vi "Add Library To Project.vi"(8 "error in":errorcluster, 10 "template folder path":path, 11 "configuration":T1) -> (0 "error out":errorcluster, 3 "project ref out":refnum<vi>)   [LabVIEW 2021, in "InstrumentStudio Plug-In Editor.lvlib"]
uses:
  InstrumentStudio Plug-In Editor.lvlib
  controls/Data Holder.ctl
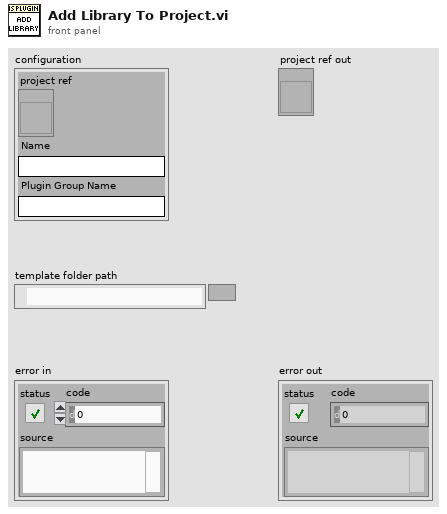
[diagram p1: front panel]
types:
  T1 = typedef "InstrumentStudio Plug-In Editor.lvlib/Data Holder.ctl" = cluster{"project ref":refnum<vi>, "Name":string, "Plugin Group Name":string}
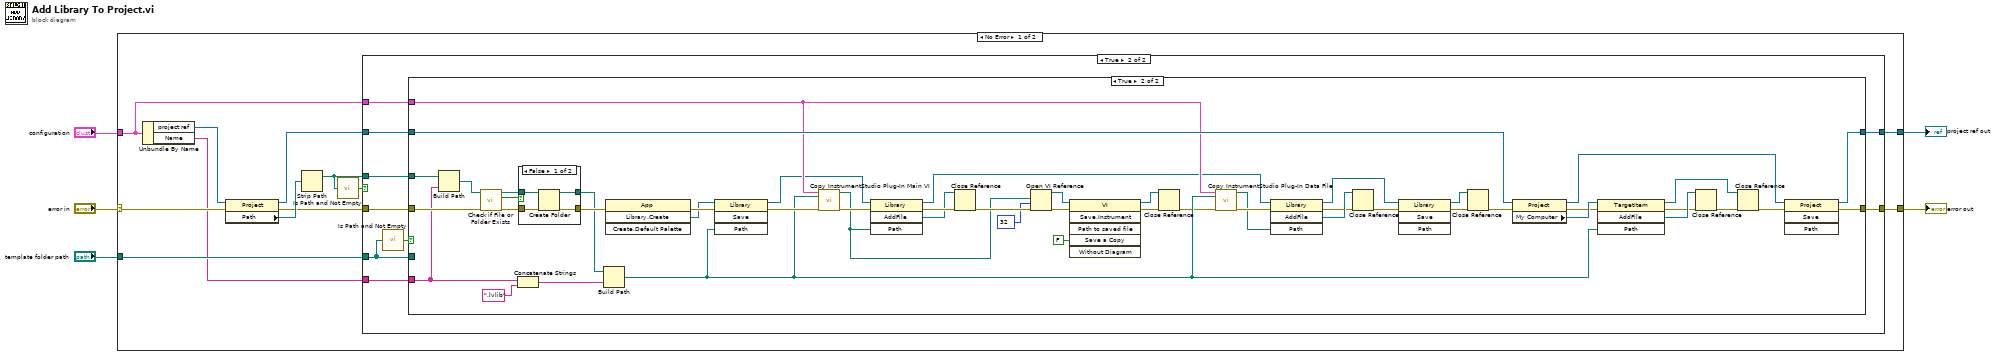
[diagram p0: block diagram]
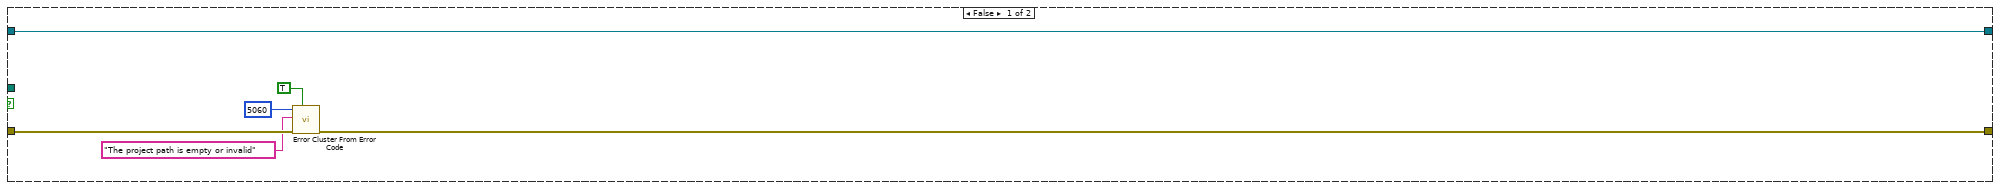
[diagram p2: hidden frame]
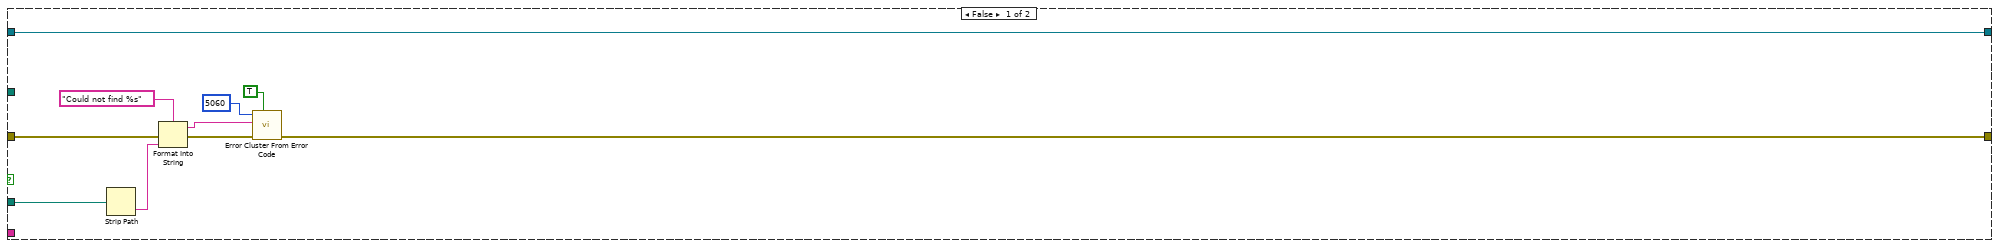
[diagram p3: hidden frame]
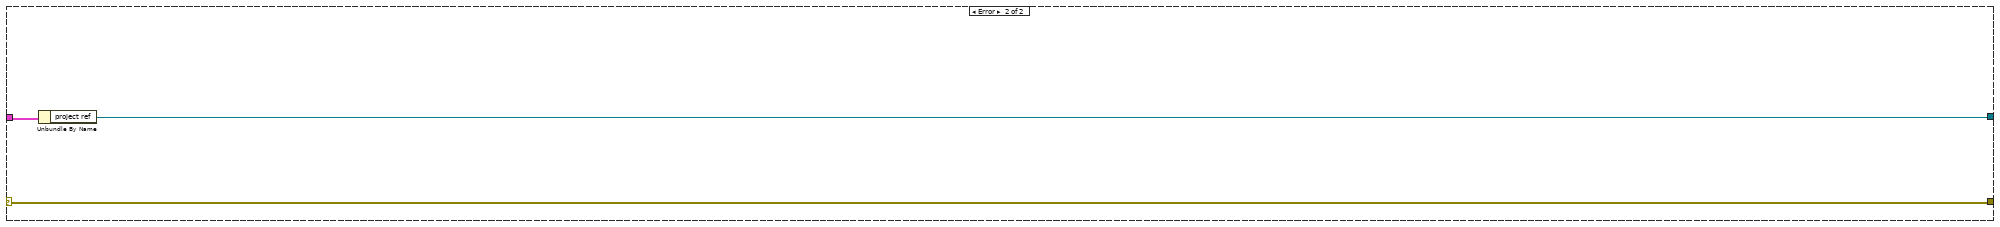
[diagram p5: hidden frame]
diagram:
  n1 = case shown="No Error" "error in" {
    selector: "error in" -> [w10 w100]
    tunnel: "template folder path" -> [w15 _]
    tunnel: [w14 w101] -> w5
    tunnel: "configuration" -> [w12 w99]
    tunnel: [w8 w100] -> w4
    frame No Error {
      n2 = Unbundle By Name(w12) -> ("project ref"=w13:refnum<vi>, "Name"=w6:string)
      n3 = property class="Project"(reference=w13, error in=w10) -> (reference out=w11:refnum<vi>, error out=w9:errorcluster, "Path"=w16:path)
      n4 = Strip Path(path=w16) -> (stripped path=w7:path)  [unwired: 1 out]
      n5 = call <vilib>:"Is Path and Not Empty.vi"("path"=w7) -> ("Is Path and Not Empty?"=w17:bool)  [unwired: 4 in]
      n6 = case shown="True" w17 {
        tunnel: w15 -> [_ w24]
        tunnel: w6 -> [_ w32]
        tunnel: w7 -> [_ w31]
        tunnel: [w23 w30] -> w14
        tunnel: w12 -> [_ w29]
        tunnel: w11 -> [w23 w28]
        tunnel: w9 -> [w22 w26]
        tunnel: [w18 w25] -> w8
        frame False {
          n7 = call <vilib>:"Error Cluster From Error Code.vi"("show call chain? (False)"=TRUE, "error in (no error)"=w22, "error message (\"\")"="The project path is empty or invalid" ("error message (\"\")"), "error code (0)"=5060) -> ("error out"=w18:errorcluster)  [unwired: 5 in]
        }
        frame True {
          n8 = call <vilib>:"Is Path and Not Empty.vi"("path"=w24) -> ("Is Path and Not Empty?"=w27:bool)  [unwired: 4 in]
          n9 = case shown="True" w27 {
            tunnel: w24 -> [w33 _]
            tunnel: w32 -> [_ w63]
            tunnel: w31 -> [_ w92]
            tunnel: [w40 w90] -> w30
            tunnel: w29 -> [_ w58]
            tunnel: w28 -> [w40 w69]
            tunnel: w26 -> [w37 w88]
            tunnel: [w34 w65] -> w25
            frame False {
              n10 = Strip Path(path=w33) -> (name=w38:string)  [unwired: 1 out]
              n11 = Format Into String(format string="Could not find %s", error in=w37, w38) -> (resulting string=w41:string, error out=w42:errorcluster)  [unwired: 1 in]
              n12 = call <vilib>:"Error Cluster From Error Code.vi"("show call chain? (False)"=TRUE, "error in (no error)"=w42, "error message (\"\")"=w41, "error code (0)"=5060) -> ("error out"=w34:errorcluster)  [unwired: 5 in]
            }
            frame True {
              n13 = Build Path(base path=w92, name or relative path=w63) -> (appended path=w91:path)
              n14 = call <vilib>:"Check if File or Folder Exists.vi"("error in (no error)"=w88, "path"=w91) -> ("error out"=w87:errorcluster, "file or folder exists?"=w85:bool, "dup path"=w86:path)  [unwired: 7 in]
              n15 = Concatenate Strings(w63, ".lvlib" ("string")) -> (w61:string)
              n16 = case shown="False" w85 {
                tunnel: w87 -> [w96 w97]
                tunnel: w86 -> [w95 w98]
                tunnel: [w94 w98] -> w62
                tunnel: [w93 w97] -> w84
                frame False {
                  n17 = Create Folder(path (use dialog)=w95, error in=w96) -> (created path=w94:path, error out=w93:errorcluster)  [unwired: 1 in, 1 out]
                }
                frame True {
                }
              }
              n18 = Build Path(base path=w62, name or relative path=w61) -> (appended path=w51:path)
              n19 = invoke class="App" method="Library.Create"(error in=w84) -> (error out=w83:errorcluster, "Create Library"=w64:refnum<vi>)  [unwired: 3 in, 2 out]
              n20 = invoke class="Library" method="Save"(reference=w64, error in=w83, "Path"=w51) -> (reference out=w56:refnum<vi>, error out=w82:errorcluster)  [unwired: 1 in, 2 out]
              n21 = call "Copy InstrumentStudio Plug-In Main VI.vi"("configuration"=w58, "Plugin Library Path"=w51, "error in"=w82) -> ("IS Plugin Main VI Path"=w49:path, "error out"=w59:errorcluster)  [unwired: 11 in]
              n22 = invoke class="Library" method="AddFile"(reference=w56, error in=w59, "Path"=w49) -> (reference out=w53:refnum<vi>, error out=w57:errorcluster, "AddFile"=w54:refnum<vi>)  [unwired: 1 in, 1 out]
              n23 = Close Reference(reference=w54, error in (no error)=w57) -> (error out=w55:errorcluster)
              n24 = Open VI Reference(vi path=w49, options=32, error in (no error)=w55) -> (vi reference=w45:refnum<vi>, error out=w50:errorcluster)  [unwired: 3 in]
              n25 = invoke class="VI" method="Save.Instrument"(reference=w45, error in=w50, "Save a Copy"=FALSE) -> (reference out=w43:refnum<vi>, error out=w47:errorcluster)  [unwired: 3 in, 4 out]
              n26 = Close Reference(reference=w43, error in (no error)=w47) -> (error out=w44:errorcluster)
              n27 = call "Copy InstrumentStudio Plug-In Data File.vi"("configuration"=w58, "Plugin Library Path"=w51, "error in"=w44) -> ("IS Plugin Data File Path"=w52:path, "error out"=w81:errorcluster)  [unwired: 11 in]
              n28 = invoke class="Library" method="AddFile"(reference=w53, error in=w81, "Path"=w52) -> (reference out=w77:refnum<vi>, error out=w79:errorcluster, "AddFile"=w89:refnum<vi>)  [unwired: 1 in, 1 out]
              n29 = Close Reference(reference=w89, error in (no error)=w79) -> (error out=w80:errorcluster)
              n30 = invoke class="Library" method="Save"(reference=w77, error in=w80) -> (reference out=w76:refnum<vi>, error out=w78:errorcluster)  [unwired: 2 in, 2 out]
              n31 = Close Reference(reference=w76, error in (no error)=w78) -> (error out=w71:errorcluster)
              n32 = property class="Project"(reference=w69, error in=w71) -> (reference out=w66:refnum<vi>, error out=w73:errorcluster, "My Computer"=w75:refnum<vi>)
              n33 = invoke class="TargetItem" method="AddFile"(reference=w75, error in=w73, "Path"=w51) -> (reference out=w67:refnum<vi>, error out=w72:errorcluster, "AddFile"=w74:refnum<vi>)  [unwired: 1 in, 1 out]
              n34 = Close Reference(reference=w74, error in (no error)=w72) -> (error out=w70:errorcluster)
              n35 = Close Reference(reference=w67, error in (no error)=w70) -> (error out=w68:errorcluster)
              n36 = invoke class="Project" method="Save"(reference=w66, error in=w68) -> (reference out=w90:refnum<vi>, error out=w65:errorcluster)  [unwired: 2 in, 2 out]
            }
          }
        }
      }
    }
    frame Error {
      n37 = Unbundle By Name(w99) -> ("project ref"=w101:refnum<vi>)
    }
  }
  "error out" <- w4
  "project ref out" <- w5
